vi "Read Channel names.vi"(8 "error in (no error)":errorcluster, 11 "Scaled I32 Array Result in":refnum<class "Scaled I32 Array Result.lvclass">) -> (0 "error out":errorcluster, 2 "Channel names":string[](array[string]), 3 "Scaled I32 Array Result out":refnum<class "Scaled I32 Array Result.lvclass">)   [LabVIEW 2015, in "Scaled I32 Array Result.lvclass"]
uses:
  Scaled I32 Array Result.lvclass
  Scaled I32 Array Result.lvclass/Scaled I32 Array Result.ctl
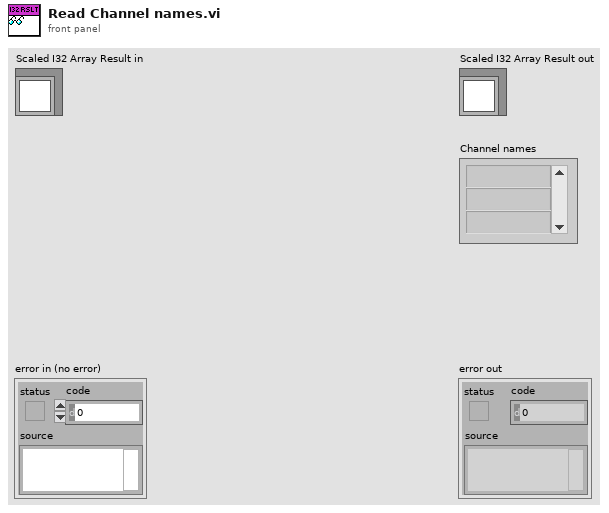
[diagram p1: front panel]
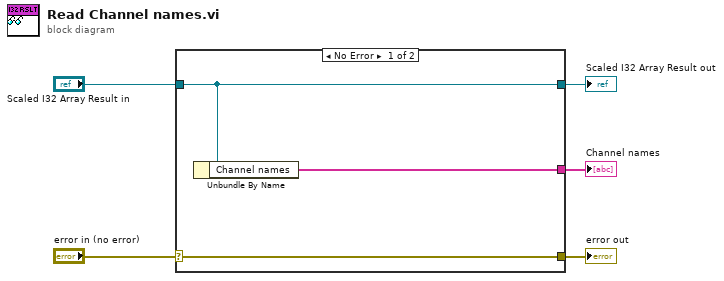
[diagram p0: block diagram]
diagram:
  n1 = case shown="No Error" "error in (no error)" {
    selector: "error in (no error)" -> [w8 w9]
    tunnel: [w8 w9] -> w4
    tunnel: [w7 w10] -> w2
    tunnel: "Scaled I32 Array Result in" -> [w7 w10]
    tunnel: [w6 _] -> w1
    frame No Error {
      n2 = Unbundle By Name(w7) -> ("Channel names"=w6:string[])
    }
    frame Error {
    }
  }
  "error out" <- w4
  "Scaled I32 Array Result out" <- w2
  "Channel names" <- w1
